vi "Rerouting.vi"(4 "Eye Model Cluster":T3={"X Grid"=[], "Y Grid"=[], "Za_true Surf"=[], "Iris Center"=[], "Zp_true Surf"=[], "Pinv"=[[1.0, 0.0], [0.0, 1.0]], "za_true"=5.0, "za_work"=1.0, "zp_work"=-1.0, "zp_true"=-5.0}, 5 "Trajectory Cluster":T1, 6 "PID Cluster":T6={"L1 to L4 PID Cluster"={"L1 PID Gains"={"Kp"=0.005, "Kd"=0.5, "Ki"=0.0005}, "L2 PID Gains"={"Kp"=0.01, "Kd"=1.0, "Ki"=0.005}, "L3 PID Gains"={"Kp"=0.05, "Kd"=1.0, "Ki"=0.0005}, "L4 PID Gains"={"Kp"=0.1, "Kd"=0.1, "Ki"=0.0005}}, "Stage PID Cluster"={"Stage Z PID"={"Kp"=0.0005, "Kd"=0.001, "Ki"=0.0}, "Stage Y PID"={"Kp"=0.0003, "Kd"=0.01, "Ki"=0.0}, "Stage X PID"={"Kp"=0.0003, "Kd"=0.01, "Ki"=0.0}}, "OCT Z PID Gains"={"Kp"=0.0003, "Kd"=0.0001, "Ki"=0.01}}, 7 "Offset Home 2 RCM":dbl[](array[numeric])=[0.0, 0.0, 0.0, 0.0], 8 "error in":errorcluster, 9 "Prev Index":i32, 10 "Prev Posit Cluster":T5={"Prev L1 to L4 Posit"=[-0.5319, -0.035669172703475985, -2.0566170657346783, 0.9099264705882353], "Prev Stage Posit"=[6.002553885707208, 5.996566124542428, 5.995469940427586], "Prev OCT Z Posit"=-0.0}, 11 "FPGA VI Reference In":refnum<k20>) -> (0 "error out":errorcluster, 1 "Last Index":i32, 2 "Last Posit Cluster":T4={"Last L1 to L4 Posit"=[0.0, 0.0, 0.0, 0.0], "Last Stage Posit"=[6.0, 6.0, 6.0], "Last OCT Z Posit"=0.0}, 3 "FPGA VI Reference Out":refnum<k20>)   [LabVIEW 2016]
uses:
  <vilib>/Analysis/Matrix/Datatypes/RealMatrix.ctl
  <vilib>/Platform/TimedLoop/XDataNode/timing_clust.ctl
  <vilib>/Platform/TimedLoop/XDataNode/nitl_modes.ctl
  <vilib>/Platform/TimedLoop/XDataNode/wakeup.ctl
  <vilib>/Analysis/_algsub.llb/Vector Norm Type.ctl
  <vilib>/Analysis/_algsub.llb/Real Vector Norm.vi
  Global Variables.vi
  <vilib>/platform/TimedLoop/XDataNode/XDataNode.xnode
  <vilib>/Platform/TimedLoop/XDataNode/XDNodeRunTimeDep.lvlib
  <vilib>/Analysis/NI_AALPro.lvlib
  <vilib>/Analysis/Matrix/NI_Matrix.lvlib
panel:
  out "In Servo Loop":bool
  out "Calc Finished":bool
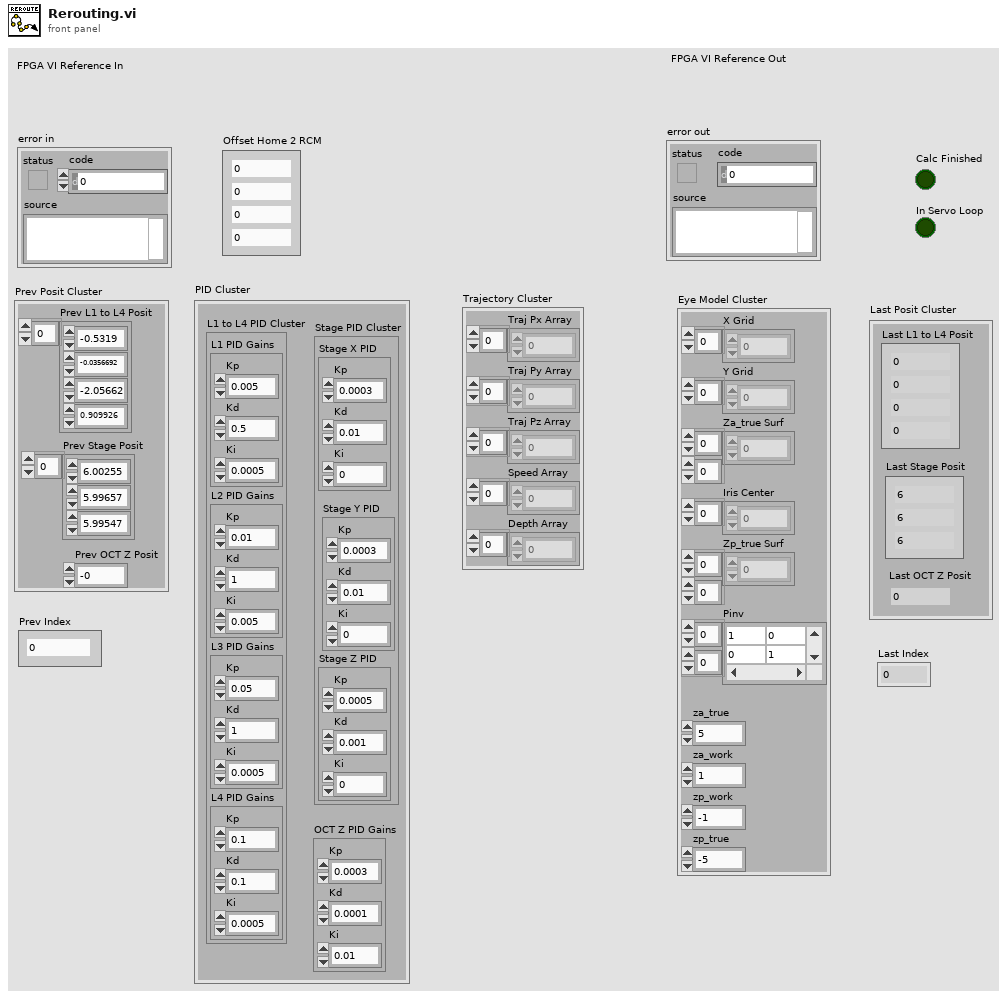
[diagram p1: front panel]
types:
  T1 = cluster{"Traj Px Array":dbl[], "Traj Py Array":dbl[], "Traj Pz Array":dbl[], "Speed Array":dbl[], "Depth Array":dbl[]}
  T2 = typedef "NI_Matrix.lvlib/RealMatrix.ctl" = dbl[][]
  T3 = cluster{"X Grid":dbl[], "Y Grid":dbl[], "Za_true Surf":dbl[][], "Iris Center":dbl[], "Zp_true Surf":dbl[][], "Pinv":T2, "za_true":dbl, "za_work":dbl, "zp_work":dbl, "zp_true":dbl}
  T4 = cluster{"Last L1 to L4 Posit":dbl[], "Last Stage Posit":dbl[], "Last OCT Z Posit":dbl}
  T5 = cluster{"Prev L1 to L4 Posit":dbl[], "Prev Stage Posit":dbl[], "Prev OCT Z Posit":dbl}
  T6 = cluster{"L1 to L4 PID Cluster":cluster{"L1 PID Gains":cluster{"Kp":dbl, "Kd":dbl, "Ki":dbl}, "L2 PID Gains":cluster{"Kp":dbl, "Kd":dbl, "Ki":dbl}, "L3 PID Gains":cluster{"Kp":dbl, "Kd":dbl, "Ki":dbl}, "L4 PID Gains":cluster{"Kp":dbl, "Kd":dbl, "Ki":dbl}}, "Stage PID Cluster":cluster{"Stage Z PID":cluster{"Kp":dbl, "Kd":dbl, "Ki":dbl}, "Stage Y PID":cluster{"Kp":dbl, "Kd":dbl, "Ki":dbl}, "Stage X PID":cluster{"Kp":dbl, "Kd":dbl, "Ki":dbl}}, "OCT Z PID Gains":cluster{"Kp":dbl, "Kd":dbl, "Ki":dbl}}
  T7 = typedef "XDNodeRunTimeDep.lvlib/timing_clust.ctl" = cluster{"Expected End [f-1]":u64, "Actual End [f-1]":u64, "Finished Late? [f-1]":bool, "Expected End [i-1]":u64, "Actual End [i-1]":u64, "Finished Late? [i-1]":bool, "Expected Start [i]":u64, "Actual Start [i]":u64, "Expected Start [f]":u64, "Actual Start [f]":u64, "Source Name":string, "Structure Name":string, "Period":i64, "Deadline":i64, "Offset":i64, "Start":i64, "Priority":i32, "Timeout":i32, "Mode":T8, "Wakeup Reason":T9, "Error":errorcluster, "Source Type":string, "Secondary Source Type":string, "Global End Time":u64, "Global Start Time":u64, "Frame Duration":u64, "Iteration Duration":u64, "Assigned CPU":i32, "I/O Scan Engine Mode":u32}
  T8 = typedef "XDNodeRunTimeDep.lvlib/nitl_modes.ctl" = enum32{"No Change", "Process missed periods, maintain original phase", "Discard missed periods, maintain original phase", "Process missed periods, ignore original phase", "Discard missed periods, ignore original phase"}
  T9 = typedef "XDNodeRunTimeDep.lvlib/wakeup.ctl" = enum32{"Normal", "Aborted", "Asynchronous wakeup", "Timing source error", "Timed loop error", "Timeout"}
  T10 = cluster{"Stop Vacuum":bool, "Vacuum Force":i8, "Max Limit [mmHg]":dbl, "Slide in":i8, "Irrigation?":bool}
  T11 = cluster{"L1 PID Gains":cluster{"Kp":dbl, "Kd":dbl, "Ki":dbl}, "L2 PID Gains":cluster{"Kp":dbl, "Kd":dbl, "Ki":dbl}, "L3 PID Gains":cluster{"Kp":dbl, "Kd":dbl, "Ki":dbl}, "L4 PID Gains":cluster{"Kp":dbl, "Kd":dbl, "Ki":dbl}}
  T12 = cluster{"Stage Z PID":cluster{"Kp":dbl, "Kd":dbl, "Ki":dbl}, "Stage Y PID":cluster{"Kp":dbl, "Kd":dbl, "Ki":dbl}, "Stage X PID":cluster{"Kp":dbl, "Kd":dbl, "Ki":dbl}}
  T13 = cluster{"Accurus button":bool[], "Accurus engaged?":bool, "Vacuum Force":i32, "Accurus Ch. A Vout":dbl, "Accurus Ch. B Vout":dbl, "Irrigation engaged?":bool}
  T14 = typedef "NI_AALPro.lvlib/Vector Norm Type.ctl" = u16
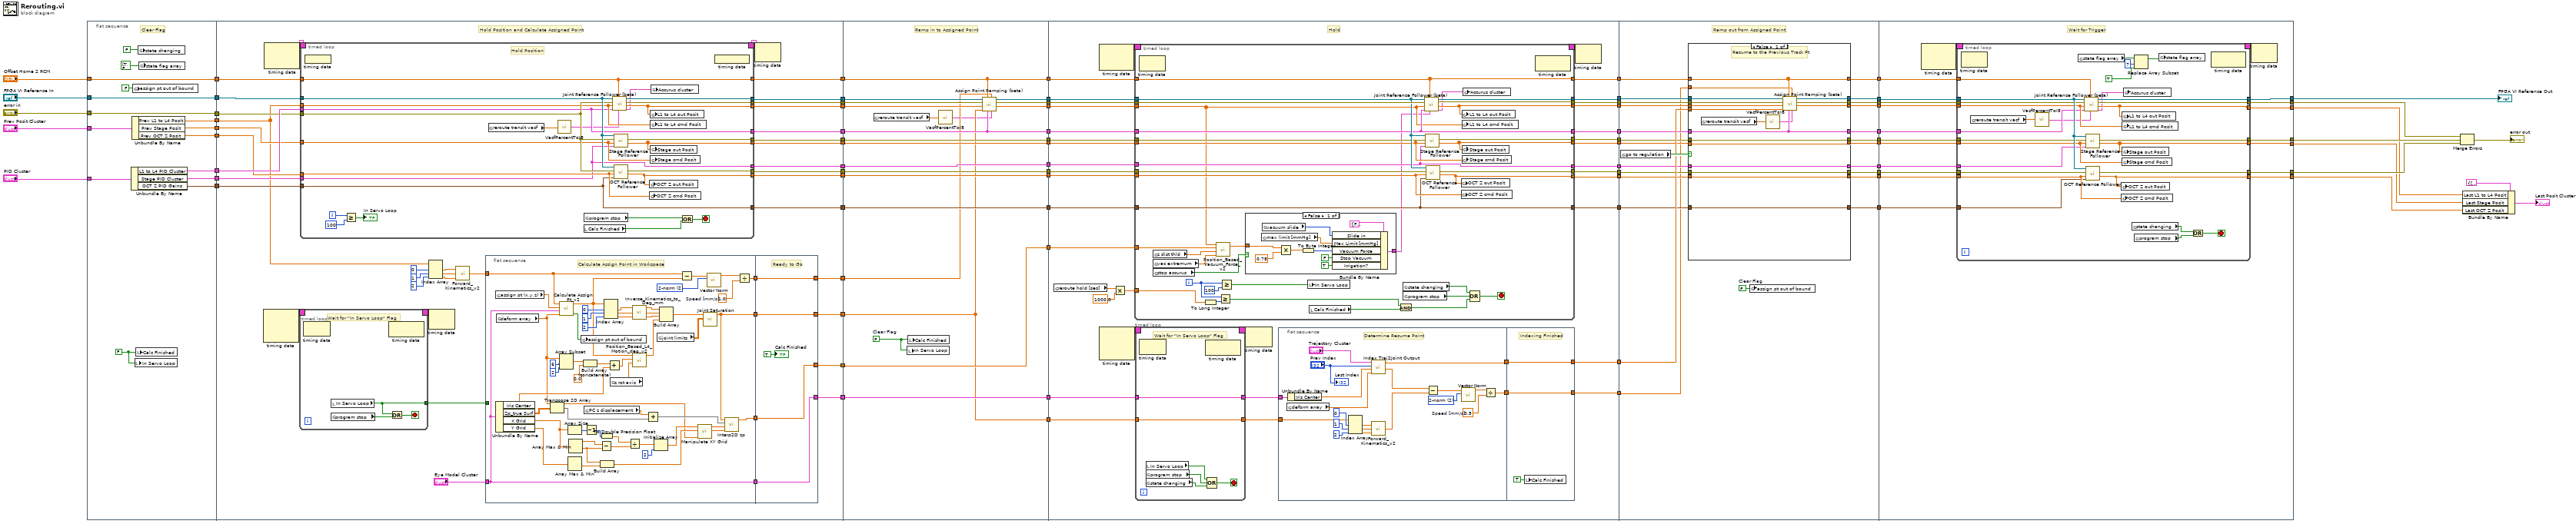
[diagram p0: block diagram]
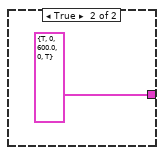
[diagram p2: hidden frame]
diagram:
  n1 = flat-sequence {
    tunnel: [w90] -> w77
    tunnel: "FPGA VI Reference In" -> [w90]
    tunnel: [w89] -> w75
    tunnel: "error in" -> [w89]
    tunnel: "Prev Posit Cluster" -> [w88]
    tunnel: "PID Cluster" -> [w87]
    tunnel: [w86] -> w73
    tunnel: [w85] -> w72
    tunnel: "Offset Home 2 RCM" -> [w84]
    tunnel: [w84] -> w70
    tunnel: [w83] -> w67
    tunnel: [w82] -> w66
    tunnel: [w81] -> w65
    tunnel: [w80] -> w64
    tunnel: w77 -> [w120]
    tunnel: w75 -> [w116]
    tunnel: w73 -> [w118]
    tunnel: w72 -> [w117]
    tunnel: w70 -> [w121]
    tunnel: w67 -> [w106]
    tunnel: w66 -> [w115]
    tunnel: w65 -> [w114]
    tunnel: w64 -> [w119]
    tunnel: [w133] -> w53
    tunnel: [w132] -> w52
    tunnel: [w131] -> w51
    tunnel: [w130] -> w50
    tunnel: [w129] -> w49
    tunnel: [w128] -> w48
    tunnel: [w127] -> w47
    tunnel: [w126] -> w46
    tunnel: [w113] -> w45
    tunnel: [w112] -> w44
    tunnel: [w111] -> w43
    tunnel: [w101] -> w8
    tunnel: [w97] -> w6
    tunnel: [w95] -> w5
    tunnel: [w93] -> w3
    tunnel: w53 -> [w240]
    tunnel: [w239] -> w42
    tunnel: w52 -> [w241]
    tunnel: [w241] -> w41
    tunnel: w51 -> [w232]
    tunnel: [w236] -> w40
    tunnel: w50 -> [w247]
    tunnel: [w247] -> w39
    tunnel: w49 -> [w246]
    tunnel: [w246] -> w38
    tunnel: w48 -> [w245]
    tunnel: [w245] -> w37
    tunnel: w47 -> [w235]
    tunnel: [w235] -> w36
    tunnel: w46 -> [w244]
    tunnel: [w244] -> w35
    tunnel: w45 -> [w238]
    tunnel: [w237] -> w34
    tunnel: w44 -> [w243]
    tunnel: [w243] -> w33
    tunnel: w43 -> [w242]
    tunnel: [w242] -> w32
    tunnel: [w233] -> w9
    tunnel: w8 -> [w233]
    tunnel: w6 -> [w229]
    tunnel: w5 -> [w231]
    tunnel: [w231] -> w4
    tunnel: w3 -> [w230]
    tunnel: [w229] -> w1
    tunnel: w42 -> [w282]
    tunnel: [w278] -> w31
    tunnel: w41 -> [w283]
    tunnel: [w269] -> w29
    tunnel: w40 -> [w280]
    tunnel: [w268] -> w27
    tunnel: w39 -> [w273]
    tunnel: [w266] -> w25
    tunnel: w38 -> [w271]
    tunnel: [w265] -> w23
    tunnel: w37 -> [w270]
    tunnel: [w263] -> w21
    tunnel: w36 -> [w279]
    tunnel: [w267] -> w19
    tunnel: w35 -> [w272]
    tunnel: [w262] -> w17
    tunnel: w34 -> [w281]
    tunnel: [w277] -> w15
    tunnel: w33 -> [w274]
    tunnel: [w264] -> w13
    tunnel: w32 -> [w275]
    tunnel: [w276] -> w11
    tunnel: w9 -> [w258]
    tunnel: [w259] -> w7
    tunnel: w4 -> [w255]
    tunnel: [w253] -> w2
    tunnel: w1 -> [w252]
    tunnel: w31 -> [w393]
    tunnel: [w388] -> w30
    tunnel: w29 -> [w394]
    tunnel: [w372] -> w28
    tunnel: w27 -> [w391]
    tunnel: [w386] -> w26
    tunnel: w25 -> [w382]
    tunnel: [w381] -> w24
    tunnel: w23 -> [w376]
    tunnel: [w375] -> w22
    tunnel: w21 -> [w374]
    tunnel: [w373] -> w20
    tunnel: w19 -> [w389]
    tunnel: [w383] -> w18
    tunnel: w17 -> [w380]
    tunnel: [w379] -> w16
    tunnel: w15 -> [w392]
    tunnel: [w387] -> w14
    tunnel: w13 -> [w377]
    tunnel: [w378] -> w12
    tunnel: w11 -> [w384]
    tunnel: [w385] -> w10
    tunnel: w7 -> [w390]
    tunnel: w2 -> [w370]
    tunnel: w30 -> [w442]
    tunnel: [w441] -> w62
    tunnel: [w440] -> w61
    tunnel: [w439] -> w60
    tunnel: w28 -> [w438]
    tunnel: w26 -> [w437]
    tunnel: w24 -> [w436]
    tunnel: w22 -> [w435]
    tunnel: w20 -> [w434]
    tunnel: w18 -> [w433]
    tunnel: w16 -> [w432]
    tunnel: [w431] -> w58
    tunnel: [w430] -> w57
    tunnel: [w429] -> w56
    tunnel: [w428] -> w54
    tunnel: w14 -> [w427]
    tunnel: w12 -> [w426]
    tunnel: w10 -> [w425]
    frame #0 {
      w79 = FALSE ("Loading Finished")
      # "Clear Flag"
      n2 = Unbundle By Name(w87) -> ("L1 to L4 PID Cluster"=w85:T11, "Stage PID Cluster"=w86:T12, "OCT Z PID Gains"=w80:cluster{"Kp":dbl, "Kd":dbl, "Ki":dbl})
      n3 = Unbundle By Name(w88) -> ("Prev L1 to L4 Posit"=w83:dbl[], "Prev Stage Posit"=w82:dbl[], "Prev OCT Z Posit"=w81:dbl)
      n4 = global write "Global Variables.vi" "assign pt out of bound"(FALSE ("assign pt out of bound")) -> ()
      n5 = local write "In Servo Loop"(w79) -> ()
      n6 = local write "Calc Finished"(w79) -> ()
      n7 = global write "Global Variables.vi" "state changing"(FALSE ("state changing")) -> ()
      n8 = global write "Global Variables.vi" "state flag array"(bool[] [TRUE, FALSE, FALSE, FALSE, FALSE, FALSE, FALSE, FALSE, FALSE] ("state flag array")) -> ()
    }
    frame #1 {
      # "Hold Position and Calculate Assigned Point"
      n9 = node-c288() -> (w123:T7)  [unwired: 3 in]
      n10 = node-c288() -> (w125:T7)  [unwired: 2 in]
      n11 = timed-loop {
        timing: w123 -> [_]
        timing-out: [_] -> w122
        tunnel: [w191] -> w99
        stop <- w193 stop-if-true
        # "Wait for \"In Servo Loop\" Flag"
        n12 = node-c288() -> ()  [unwired: 1 in, 1 out]
        n13 = global read "Global Variables.vi" "program stop"() -> (w192:bool)
        n14 = local read "In Servo Loop"() -> (w191:bool)
        n15 = node-c288() -> ()  [unwired: 1 in, 1 out]
        n16 = Or(x=w191, y=w192) -> (x .or. y?=w193:bool)
      }
      n17 = timed-loop {
        timing: w125 -> [_]
        timing-out: [_] -> w124
        tunnel: w106 -> [w216]
        tunnel: w115 -> [w214]
        tunnel: w118 -> [w204]
        tunnel: w117 -> [w205]
        tunnel: w116 -> [w218]
        tunnel: w120 -> [w219]
        tunnel: w121 -> [w211]
        tunnel: w114 -> [w212]
        tunnel: w119 -> [w206]
        tunnel: [w217] -> w131
        tunnel: [w215] -> w130
        tunnel: [w213] -> w129
        tunnel: [w211] -> w132
        tunnel: [w210] -> w133
        tunnel: [w209] -> w113
        tunnel: [w208] -> w111
        tunnel: [w207] -> w112
        tunnel: [w206] -> w128
        tunnel: [w205] -> w127
        tunnel: [w204] -> w126
        i -> [w203]
        stop <- w222 stop-if-true
        # "Hold Position"
        n18 = node-c288 ("Output Node")() -> ()  [unwired: 1 in]
        n19 = Greater Or Equal?(x=w203, y=100) -> (x >= y?=→"In Servo Loop":bool)
        n20 = global read "Global Variables.vi" "reroute transit vacf"() -> (w199:dbl)
        n21 = call "VacfPercentToI8.vi"("vacf (0-100)"=w199) -> ("Accurus Ctrl Cluster"=w198:T10)
        n22 = local read "Calc Finished"() -> (w221:bool)
        n23 = global read "Global Variables.vi" "program stop"() -> (w220:bool)
        n24 = call "Joint Reference Follower (beta).vi"("Accurus Ctrl Cluster"=w198, "Offset Home2RCM [deg/mm]"=w211, "PID Ctrl Cluster"=w205, "Ref Array [deg/mm]"=w216, "error in"=w218, "FPGA VI Reference In"=w219) -> ("Accurus Output Cluster"=w200:T13, "Output Posit Array [deg/mm]"=w217:dbl[], "error out"=w209:errorcluster, "FPGA VI Reference Out"=w210:refnum<k20>)  [unwired: 2 in]
        n25 = call "Stage Reference Follower.vi"("Stage PID Cluster"=w204, "Stage cmd Posit [mm]"=w214, "error in"=w218, "FPGA VI Reference In"=w219) -> ("Stage out Posit [mm]"=w215:dbl[], "error out"=w208:errorcluster)  [unwired: 5 in, 1 out]
        n26 = call "OCT Reference Follower.vi"("OCT Z PID Gains"=w206, "OCT  Z cmd Posit [mm]"=w212, "error in"=w218, "FPGA VI Reference In"=w219) -> ("OCT  Z out Posit [mm]"=w213:dbl, "error out"=w207:errorcluster)  [unwired: 5 in, 1 out]
        n27 = global write "Global Variables.vi" "OCT Z out Posit"(w213) -> ()
        n28 = global write "Global Variables.vi" "OCT Z cmd Posit"(w212) -> ()
        n29 = global write "Global Variables.vi" "L1 to L4 out Posit"(w217) -> ()
        n30 = global write "Global Variables.vi" "L1 to L4 cmd Posit"(w216) -> ()
        n31 = global write "Global Variables.vi" "Stage out Posit"(w215) -> ()
        n32 = global write "Global Variables.vi" "Stage cmd Posit"(w214) -> ()
        n33 = global write "Global Variables.vi" "Accurus cluster"(w200) -> ()
        n34 = Or(x=w220, y=w221) -> (x .or. y?=w222:bool)
        n35 = node-c288() -> ()  [unwired: 1 out]
      }
      n36 = Index Array(array=w106, index #1=0 ("index"), index #2=1 ("index"), index #3=2 ("index")) -> (element #1=w109:dbl, element #2=w108:dbl, element #3=w107:dbl)
      n37 = node-c288(w122) -> ()  [unwired: 1 out]
      n38 = call "Forward_Kinematics_v2.vi"("theta 3"=w107, "theta 2"=w108, "theta 1"=w109) -> ("position"=w102:dbl[])
      n39 = flat-sequence {
        tunnel: "Eye Model Cluster" -> [w162]
        tunnel: w102 -> [w153]
        tunnel: [w162] -> w100
        tunnel: w99 -> [_]
        tunnel: [w135] -> w98
        tunnel: [w154] -> w96
        tunnel: [w148] -> w94
        tunnel: [w189] -> w101
        tunnel: w100 -> [w189]
        tunnel: [w188] -> w97
        tunnel: w98 -> [w188]
        tunnel: [w186] -> w95
        tunnel: w96 -> [w186]
        tunnel: [w187] -> w93
        tunnel: w94 -> [w187]
        frame #0 {
          w149 = 1.0  # Speed [mm/s]
          w151 = T14 2 items=["1-norm"=1, "2-norm"=2, "Inf-norm"=3, "-Inf-norm"=4, "User Defined"=5] ("norm type")
          # "Calculate Assign Point in Workspace"
          n40 = global read "Global Variables.vi" "assign pt (x,y,z)"() -> (w185:dbl[])
          n41 = Unbundle By Name(w162) -> ("Iris Center"=w139:dbl[], "Zp_true Surf"=w172:dbl[][], "X Grid"=w171:dbl[], "Y Grid"=w163:dbl[])
          n42 = global read "Global Variables.vi" "deform array"() -> (w138:dbl[])
          n43 = Transpose 2D Array(2D array=w172) -> (transposed array=w157:dbl[][])
          n44 = call "Calculate Assign Pt_v2.vi"("Deform Array"=w138, "Eye Model Cluster"=w162, "Assign Pt"=w185, "Current Pt"=w153) -> ("Assign Pt OOB"=w184:bool, "Assign Pt*"=w146:dbl[])  [unwired: 6 in]
          n45 = Array Subset(array=w138, index=6, length=2) -> (w137:dbl[])
          n46 = Array Size(array=w171) -> (size(s)=w164:i32)
          n47 = Array Max & Min(array=w163) -> (min value=w167:dbl)  [unwired: 3 out]
          n48 = Array Max & Min(array=w171) -> (max value=w166:dbl, min value=w165:dbl)  [unwired: 2 out]
          n49 = global write "Global Variables.vi" "assign pt out of bound"(w184) -> ()
          n50 = Build Array (concatenate)(w137, 0.0) -> (w143:dbl[])
          n51 = global read "Global Variables.vi" "PC z displacement"() -> (w158:dbl)
          n52 = Decrement(x=w164) -> (x-1=w169:i32)
          n53 = Subtract(x=w166, y=w165) -> (x-y=w170:dbl)
          n54 = To Double Precision Float(number=w169) -> (double precision float=w168:dbl)
          n55 = Build Array(w165, w167) -> (w155:dbl[])
          n56 = Index Array(array=w146, index #1=0 ("index"), index #2=1 ("index"), index #3=2 ("index")) -> (element #1=w180:dbl, element #2=w179:dbl, element #3=w178:dbl)
          n57 = Add(x=w143, y=w139) -> (x+y=w140:dbl[])
          n58 = global read "Global Variables.vi" "z rot axis"() -> (w145:dbl)
          n59 = Divide(x=w168, y=w170) -> (x/y=w160:dbl)
          n60 = call "Inverse_Kinematics_to_Deg_mm.vi"("pz"=w178, "py"=w179, "px"=w180) -> ("L3 [mm]"=w175:dbl, "L2 [deg]"=w176:dbl, "L1 [deg]"=w177:dbl)
          n61 = call "Position_Based_L4_Motion_deg_v2.vi"("Assign z"=w145, "Iris Center"=w140, "Tip Position"=w146) -> ("L4 Motion [deg]"=w147:dbl)  [unwired: 8 in]
          n62 = Add(x=w158, y=w157) -> (x+y=w156:dbl[][])
          n63 = Initialize Array(w160, 2 ("dimension size")) -> (w159:dbl[])
          n64 = global read "Global Variables.vi" "joint limits"() -> (w134:dbl[][])
          n65 = Build Array(w177, w176, w175, w147) -> (w136:dbl[])
          n66 = Subtract(x=w153, y=w146) -> (x-y=w152:dbl[])
          n67 = call "Manipulate XY Grid.vi"("Deform Array"=w138, "XY Grid min In"=w155, "XY Quant. Fact. In"=w159) -> ("XY Grid min Out"=w173:dbl[], "XY Quant. Fact. Out"=w174:dbl[])  [unwired: 7 in]
          n68 = call "Joint Saturation.vi"("Joint Bounds [Deg/mm]"=w134, "Ref Array [Deg/mm]"=w136) -> ("Sat Ref Array [Deg/mm]"=w135:dbl[])  [unwired: 9 in]
          n69 = call-poly <vilib>:"Vector Norm.vi"("norm type"=w151, "Input Vector"=w152) -> ("norm"=w150:dbl)  [unwired: 8 in, 1 out]
          n70 = call "Interp2D zp.vi"("XY Grid min"=w173, "XY Quantization Factor"=w174, "Zp array"=w156, "Tip Position"=w135) -> ("zp"=w154:dbl)  [unwired: 7 in]
          n71 = Divide(x=w150, y=w149) -> (x/y=w148:dbl)
        }
        frame #1 {
          # "Ready to Go"
          "Calc Finished" <- TRUE ("Loading Finished")
        }
      }
      n72 = node-c288(w124) -> ()  [unwired: 1 out]
    }
    frame #2 {
      w234 = FALSE  # Clear Flag
      # "Ramp in to Assigned Point"
      n73 = global read "Global Variables.vi" "reroute transit vacf"() -> (w228:dbl)
      n74 = local write "In Servo Loop"(w234) -> ()
      n75 = local write "Calc Finished"(w234) -> ()
      n76 = call "VacfPercentToI8.vi"("vacf (0-100)"=w228) -> ("Accurus Ctrl Cluster"=w227:T10)
      n77 = call "Assign Point Ramping (beta).vi"("Accurus Ctrl Cluster"=w227, "Ramp Time [sec]"=w230, "L1 to L4 PID Cluster"=w235, "Offset Home2RCM"=w241, "Destination Posit Array [mm]"=w229, "Previous Posit Array"=w232, "error in"=w238, "FPGA VI Reference In"=w240) -> ("Last L1 to L4 Posit"=w236:dbl[], "error out"=w237:errorcluster, "FPGA VI Reference Out"=w239:refnum<k20>)  [unwired: 1 in]
    }
    frame #3 {
      # "Hold"
      n78 = global read "Global Variables.vi" "reroute hold [sec]"() -> (w250:dbl)
      n79 = node-c288() -> (w285:T7)  [unwired: 2 in]
      n80 = node-c288() -> (w261:T7)  [unwired: 3 in]
      n81 = Multiply(x=w250, y=1000.0) -> (x*y=w248:dbl)
      n82 = timed-loop {
        timing: w285 -> [_]
        timing-out: [_] -> w284
        tunnel: w283 -> [w345]
        tunnel: w282 -> [w353]
        tunnel: w281 -> [w354]
        tunnel: w280 -> [w324]
        tunnel: w279 -> [w343]
        tunnel: [w352] -> w278
        tunnel: [w351] -> w277
        tunnel: [w350] -> w276
        tunnel: w275 -> [w349]
        tunnel: w274 -> [w348]
        tunnel: w273 -> [w347]
        tunnel: w272 -> [w338]
        tunnel: w271 -> [w346]
        tunnel: w270 -> [w339]
        tunnel: [w345] -> w269
        tunnel: [w344] -> w268
        tunnel: [w343] -> w267
        tunnel: [w342] -> w266
        tunnel: [w341] -> w265
        tunnel: [w340] -> w264
        tunnel: [w339] -> w263
        tunnel: [w338] -> w262
        tunnel: w255 -> [w325]
        tunnel: w248 -> [w319]
        i -> [w337]
        stop <- w330 stop-if-true
        n83 = node-c288() -> ()  [unwired: 1 in, 1 out]
        n84 = global read "Global Variables.vi" "z dist thld"() -> (w328:dbl[])
        n85 = global read "Global Variables.vi" "vac extremum"() -> (w327:dbl[])
        n86 = global read "Global Variables.vi" "stop accurus"() -> (w326:bool)
        n87 = To Long Integer(number=w319) -> (32bit integer=w320:i32)
        n88 = call "Position_Based_Vacuum_Force_v2.vi"("vac_bnd"=w327, "z_thld"=w328, "current zp"=w325, "tip position"=w324) -> ("vacf (%)"=w329:dbl)  [unwired: 7 in]
        n89 = Greater Or Equal?(x=w337, y=w320) -> (x >= y?=w334:bool)
        n90 = Greater Or Equal?(x=w337, y=100) -> (x >= y?=w336:bool)
        n91 = case shown="False" w326 {
          tunnel: [w358 T10 {"Stop Vacuum"=TRUE, "Vacuum Force"=0, "Max Limit [mmHg]"=600.0, "Slide in"=0, "Irrigation?"=TRUE} ("Accurus Ctrl Cluster")] -> w323
          tunnel: w329 -> [w357 _]
          frame False {
            n92 = global read "Global Variables.vi" "max limit [mmHg]"() -> (w362:dbl)
            n93 = global read "Global Variables.vi" "vacuum slide"() -> (w363:i8)
            n94 = Multiply(x=w357, y=0.78 ("x")) -> (x*y=w360:dbl)
            n95 = To Byte Integer(number=w360) -> (8bit integer=w359:i8)
            n96 = Bundle By Name(cluster=T10 {"Stop Vacuum"=FALSE, "Vacuum Force"=0, "Max Limit [mmHg]"=0.0, "Slide in"=0, "Irrigation?"=FALSE} ("Accurus Ctrl Cluster"), "Slide in"=w363, "Max Limit [mmHg]"=w362, "Vacuum Force"=w359, "Stop Vacuum"=FALSE ("Stop Accurus"), "Irrigation?"=TRUE) -> (w358:T10)
          }
          frame True {
          }
        }
        n97 = local write "In Servo Loop"(w336) -> ()
        n98 = local read "Calc Finished"() -> (w335:bool)
        n99 = And(x=w334, y=w335) -> (x .and. y?=w333:bool)
        n100 = global read "Global Variables.vi" "state changing"() -> (w332:bool)
        n101 = global read "Global Variables.vi" "program stop"() -> (w331:bool)
        n102 = call "Joint Reference Follower (beta).vi"("Accurus Ctrl Cluster"=w323, "Offset Home2RCM [deg/mm]"=w345, "PID Ctrl Cluster"=w343, "Ref Array [deg/mm]"=w324, "error in"=w354, "FPGA VI Reference In"=w353) -> ("Accurus Output Cluster"=w322:T13, "Output Posit Array [deg/mm]"=w344:dbl[], "error out"=w351:errorcluster, "FPGA VI Reference Out"=w352:refnum<k20>)  [unwired: 2 in]
        n103 = call "Stage Reference Follower.vi"("Stage PID Cluster"=w338, "Stage cmd Posit [mm]"=w347, "error in"=w349, "FPGA VI Reference In"=w353) -> ("Stage out Posit [mm]"=w342:dbl[], "error out"=w350:errorcluster)  [unwired: 5 in, 1 out]
        n104 = call "OCT Reference Follower.vi"("OCT Z PID Gains"=w339, "OCT  Z cmd Posit [mm]"=w346, "error in"=w348, "FPGA VI Reference In"=w353) -> ("OCT  Z out Posit [mm]"=w341:dbl, "error out"=w340:errorcluster)  [unwired: 5 in, 1 out]
        n105 = global write "Global Variables.vi" "OCT Z out Posit"(w341) -> ()
        n106 = global write "Global Variables.vi" "OCT Z cmd Posit"(w346) -> ()
        n107 = global write "Global Variables.vi" "L1 to L4 out Posit"(w344) -> ()
        n108 = global write "Global Variables.vi" "L1 to L4 cmd Posit"(w324) -> ()
        n109 = global write "Global Variables.vi" "Stage out Posit"(w342) -> ()
        n110 = global write "Global Variables.vi" "Stage cmd Posit"(w347) -> ()
        n111 = global write "Global Variables.vi" "Accurus cluster"(w322) -> ()
        n112 = Compound Arithmetic op=OR(w332, w331, w333) -> (w330:bool)
        n113 = node-c288() -> ()  [unwired: 1 in, 1 out]
      }
      n114 = timed-loop {
        timing: w261 -> [_]
        timing-out: [_] -> w260
        tunnel: w258 -> [w314]
        tunnel: [w314] -> w257
        tunnel: w252 -> [w309]
        tunnel: [w309] -> w251
        stop <- w313 stop-if-true
        # "Wait for \"In Servo Loop\" Flag"
        n115 = node-c288() -> ()  [unwired: 1 in, 1 out]
        n116 = local read "In Servo Loop"() -> (w311:bool)
        n117 = global read "Global Variables.vi" "program stop"() -> (w310:bool)
        n118 = global read "Global Variables.vi" "state changing"() -> (w312:bool)
        n119 = node-c288() -> ()  [unwired: 1 in, 1 out]
        n120 = Compound Arithmetic op=OR(w311, w310, w312) -> (w313:bool)
      }
      n121 = node-c288(w260) -> ()  [unwired: 1 out]
      n122 = flat-sequence {
        tunnel: w257 -> [w304]
        tunnel: [w294] -> w256
        tunnel: [w296] -> w254
        tunnel: w251 -> [w290]
        tunnel: w256 -> [w307]
        tunnel: [w307] -> w259
        tunnel: [w306] -> w253
        tunnel: w254 -> [w306]
        frame #0 {
          w300 = 0.5  # Speed [mm/s]
          w302 = T14 2 items=["1-norm"=1, "2-norm"=2, "Inf-norm"=3, "-Inf-norm"=4, "User Defined"=5] ("norm type")
          # "Determine Resume Point"
          n123 = global read "Global Variables.vi" "deform array"() -> (w297:dbl[])
          n124 = Unbundle By Name(w304) -> ("Iris Center"=w298:dbl[])
          n125 = Index Array(array=w290, index #1=0 ("index"), index #2=1 ("index"), index #3=2 ("index")) -> (element #1=w289:dbl, element #2=w288:dbl, element #3=w287:dbl)
          n126 = call "Index Traj2Joint Output.vi"("Deform Array"=w297, "Pivot Pt"=w298, "Index"="Prev Index", "Trajectory Cluster"="Trajectory Cluster") -> ("Indexed Cart Posit"=w295:dbl[], "Indexed Joit Posit"=w294:dbl[])  [unwired: 6 in]
          n127 = call "Forward_Kinematics_v2.vi"("theta 3"=w287, "theta 2"=w288, "theta 1"=w289) -> ("position"=w286:dbl[])
          n128 = Subtract(x=w295, y=w286) -> (x-y=w303:dbl[])
          n129 = call-poly <vilib>:"Vector Norm.vi"("norm type"=w302, "Input Vector"=w303) -> ("norm"=w301:dbl)  [unwired: 8 in, 1 out]
          n130 = Divide(x=w301, y=w300) -> (x/y=w296:dbl)
          "Last Index" <- "Prev Index"
        }
        frame #1 {
          # "Indexing Finished"
          n131 = local write "Calc Finished"(TRUE ("Calc Finished")) -> ()
        }
      }
      n132 = node-c288(w284) -> ()  [unwired: 1 out]
    }
    frame #4 {
      w371 = FALSE  # Clear Flag
      # "Ramp out from Assigned Point"
      n133 = global read "Global Variables.vi" "go to regulation"() -> (w395:bool)
      n134 = case shown="False" w395 {
        tunnel: w394 -> [w399 w424]
        tunnel: w393 -> [w413 w423]
        tunnel: w392 -> [w412 w422]
        tunnel: w391 -> [w411 w421]
        tunnel: w390 -> [w410 _]
        tunnel: w389 -> [w405 w420]
        tunnel: [w409 w423] -> w388
        tunnel: [w408 w422] -> w387
        tunnel: [w407 w421] -> w386
        tunnel: [w406 w419] -> w385
        tunnel: w384 -> [w406 w419]
        tunnel: [w405 w420] -> w383
        tunnel: [w404 w418] -> w381
        tunnel: w382 -> [w404 w418]
        tunnel: w380 -> [w403 w417]
        tunnel: [w403 w417] -> w379
        tunnel: [w402 w416] -> w378
        tunnel: w377 -> [w402 w416]
        tunnel: w376 -> [w401 w415]
        tunnel: [w401 w415] -> w375
        tunnel: [w400 w414] -> w373
        tunnel: w374 -> [w400 w414]
        tunnel: [w399 w424] -> w372
        tunnel: w370 -> [w398 _]
        frame False {
          # "Resume to the Previous Track Pt"
          n135 = global read "Global Variables.vi" "reroute transit vacf"() -> (w397:dbl)
          n136 = call "VacfPercentToI8.vi"("vacf (0-100)"=w397) -> ("Accurus Ctrl Cluster"=w396:T10)
          n137 = call "Assign Point Ramping (beta).vi"("Accurus Ctrl Cluster"=w396, "Ramp Time [sec]"=w398, "L1 to L4 PID Cluster"=w405, "Offset Home2RCM"=w399, "Destination Posit Array [mm]"=w410, "Previous Posit Array"=w411, "error in"=w412, "FPGA VI Reference In"=w413) -> ("Last L1 to L4 Posit"=w407:dbl[], "error out"=w408:errorcluster, "FPGA VI Reference Out"=w409:refnum<k20>)  [unwired: 1 in]
        }
        frame True {
          # "Bypass if \"go to regulation\" bit is True"
        }
      }
      n138 = global write "Global Variables.vi" "assign pt out of bound"(w371) -> ()
    }
    frame #5 {
      # "Wait for Trigger"
      n139 = node-c288() -> (w444:T7)  [unwired: 2 in]
      n140 = timed-loop {
        timing: w444 -> [_]
        timing-out: [_] -> w443
        tunnel: w442 -> [w465]
        tunnel: w427 -> [w464]
        tunnel: [w463] -> w440
        tunnel: [w462] -> w441
        tunnel: [w461] -> w439
        tunnel: w438 -> [w460]
        tunnel: w437 -> [w459]
        tunnel: w436 -> [w458]
        tunnel: w435 -> [w457]
        tunnel: w434 -> [w456]
        tunnel: w433 -> [w455]
        tunnel: w432 -> [w454]
        tunnel: [w453] -> w431
        tunnel: [w452] -> w430
        tunnel: [w451] -> w429
        tunnel: [w450] -> w428
        tunnel: w426 -> [w449]
        tunnel: w425 -> [w448]
        stop <- w472 stop-if-true
        n141 = node-c288() -> ()  [unwired: 1 in, 1 out]
        n142 = global read "Global Variables.vi" "reroute transit vacf"() -> (w446:dbl)
        n143 = call "VacfPercentToI8.vi"("vacf (0-100)"=w446) -> ("Accurus Ctrl Cluster"=w445:T10)
        n144 = global read "Global Variables.vi" "state flag array"() -> (w469:bool[])
        n145 = call "Joint Reference Follower (beta).vi"("Accurus Ctrl Cluster"=w445, "Offset Home2RCM [deg/mm]"=w460, "PID Ctrl Cluster"=w455, "Ref Array [deg/mm]"=w459, "error in"=w464, "FPGA VI Reference In"=w465) -> ("Accurus Output Cluster"=w447:T13, "Output Posit Array [deg/mm]"=w453:dbl[], "error out"=w463:errorcluster, "FPGA VI Reference Out"=w450:refnum<k20>)  [unwired: 2 in]
        n146 = call "Stage Reference Follower.vi"("Stage PID Cluster"=w454, "Stage cmd Posit [mm]"=w458, "error in"=w448, "FPGA VI Reference In"=w465) -> ("Stage out Posit [mm]"=w452:dbl[], "error out"=w462:errorcluster)  [unwired: 5 in, 1 out]
        n147 = call "OCT Reference Follower.vi"("OCT Z PID Gains"=w456, "OCT  Z cmd Posit [mm]"=w457, "error in"=w449, "FPGA VI Reference In"=w465) -> ("OCT  Z out Posit [mm]"=w451:dbl, "error out"=w461:errorcluster)  [unwired: 5 in, 1 out]
        n148 = global write "Global Variables.vi" "OCT Z out Posit"(w451) -> ()
        n149 = global write "Global Variables.vi" "OCT Z cmd Posit"(w457) -> ()
        n150 = global write "Global Variables.vi" "L1 to L4 out Posit"(w453) -> ()
        n151 = global write "Global Variables.vi" "L1 to L4 cmd Posit"(w459) -> ()
        n152 = global write "Global Variables.vi" "Stage out Posit"(w452) -> ()
        n153 = global write "Global Variables.vi" "Stage cmd Posit"(w458) -> ()
        n154 = global write "Global Variables.vi" "Accurus cluster"(w447) -> ()
        n155 = global read "Global Variables.vi" "state changing"() -> (w471:bool)
        n156 = Replace Array Subset(array=w469, new element=TRUE ("new element/subarray"), index=7) -> (w468:bool[])
        n157 = global read "Global Variables.vi" "program stop"() -> (w470:bool)
        n158 = global write "Global Variables.vi" "state flag array"(w468) -> ()
        n159 = Or(x=w471, y=w470) -> (x .or. y?=w472:bool)
        n160 = node-c288() -> ()  [unwired: 1 in, 1 out]
      }
      n161 = node-c288(w443) -> ()  [unwired: 1 out]
    }
  }
  n162 = Merge Errors(w61, w62, w60) -> (→"error out":errorcluster)
  n163 = Bundle By Name(cluster=T4 {"Last L1 to L4 Posit"=[0.0, 0.0, 0.0, 0.0], "Last Stage Posit"=[6.0, 6.0, 6.0], "Last OCT Z Posit"=0.0} ("Last Posit Cluster 2"), "Last L1 to L4 Posit"=w58, "Last Stage Posit"=w57, "Last OCT Z Posit"=w56) -> (→"Last Posit Cluster":T4)
  "FPGA VI Reference Out" <- w54
